vi "OSA_example_acquisition.vi"() -> ()   [LabVIEW 2010]
doc: "Simple example GUI for single asynchronous acquisition of spectrum with datareduction plotting functions. \n\nWhen creating custom dataacquisition applications displaying data; copy the graphs in this example, create corresponding graph references and connect to the init vi, see example diagram."
uses:
  _OSA_class/typeDef/resolution.ctl
  _OSA_class/typeDef/sensitivityMode.ctl
  _misc/Thorlabs_FTS_misc.llb/channels_table.ctl
  _misc/Thorlabs_FTS_misc.llb/channelType_spectrum.ctl
  _OSA_class/misc_examples/example_action.ctl
  _misc/Thorlabs_FTS_misc.llb/OSA_virtualModel.ctl
  _misc/Thorlabs_FTS_misc.llb/OSA_virtualSource_RS.ctl
  _OSA_class/typeDef/acq_dataType.ctl
  _OSA_class/OSA.lvclass
  OSA20X_misc.lvlib
panel:
  in  "virtual OSA":bool
  in  "spectrum channel type":T1
  in  "channels":T2
  in  "ZOOM OUT BUTTON":bool
  in  "PANE RIGHT":bool
  in  "PANE LEFT":bool
  in  "ZOOM RESTORE":bool
  in  "ZOOM IN BUTTON":bool
  in  "single acq butt":bool
  out "Intensity Graph spectrum":i32[][](graph)
  in  "sensitivity":T3=3 items=["low", "medium low", "medium high", "high"]
  in  "exit butt":bool
  in  "resolution":T4 items=["low", "high"]
  out "waveNrMax":sgl format="%.2f"
  out "waveNrMin":sgl format="%.2f"
  out "OSA":string
  # "Right click to autoscale Y"
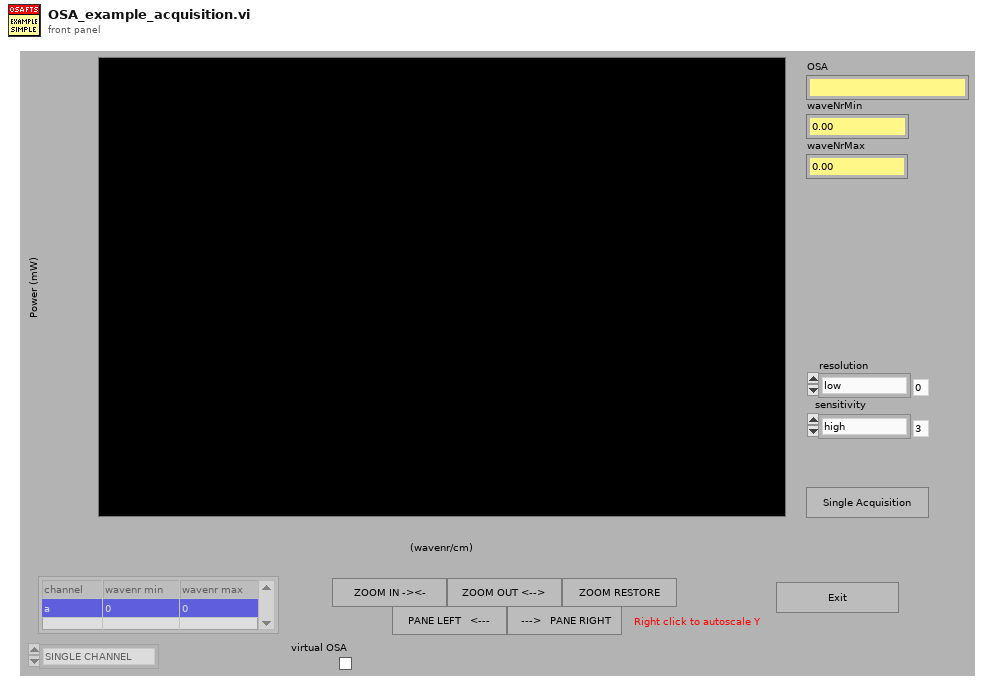
[diagram p1: front panel]
types:
  T1 = typedef "OSA20X_misc.lvlib/channelType_spectrum.ctl" = enum16{"SINGLE CHANNEL", "STICHED"}
  T2 = typedef "OSA20X_misc.lvlib/channels_table.ctl" = i32
  T3 = typedef "OSA.lvclass/sensitivityMode.ctl" = u16
  T4 = typedef "OSA.lvclass/resolution.ctl" = u16
  T5 = typedef "OSA20X_misc.lvlib/OSA_virtualSource_RS.ctl" = enum16{"VIRTUAL_REDSTONE_SOURCE_UNKNOWN", "VIRTUAL_REDSTONE_SOURCE_LLD_DFB_1530", "VIRTUAL_REDSTONE_SOURCE_SLD_1550nm", "VIRTUAL_REDSTONE_SOURCE_LASER_4600nm", "VIRTUAL_REDSTONE_SOURCE_BLACKBODY1500K", "VIRTUAL_REDSTONE_SOURCE_BLACKBODY1500K_H2O"}
  T6 = cluster{"OSA200":cluster{"waveCenter (nm)":dbl, "FWHM (nm)":dbl, "peakAmplitude":dbl}, "OSA300":T5}
  T7 = typedef "OSA20X_misc.lvlib/OSA_virtualModel.ctl" = enum16{"OSA201", "OSA201C", "OSA202", "OSA202C", "OSA203", "OSA203B", "OSA203C", "OSA205", "OSA205C", "REDSTONE301", "REDSTONE305"}
  T8 = typedef "OSA.lvclass/example_action.ctl" = enum16{"init", "user", "channel", "resolution set", "sensitivity set", "getSpectrum", "plotSpectrum"}
  T9 = cluster{"sensitivity ":refnum<vi>, "resolution":refnum<vi>, "channels":refnum<vi>, "spectrum channel type":refnum<vi>, "single acq butt":refnum<vi>}
  T10 = typedef "OSA.lvclass/acq_dataType.ctl" = enum16{"none", "interferogram", "spectrum"}
  T11 = enum8{"Enabled", "Disabled", "Disabled and Grayed Out"}
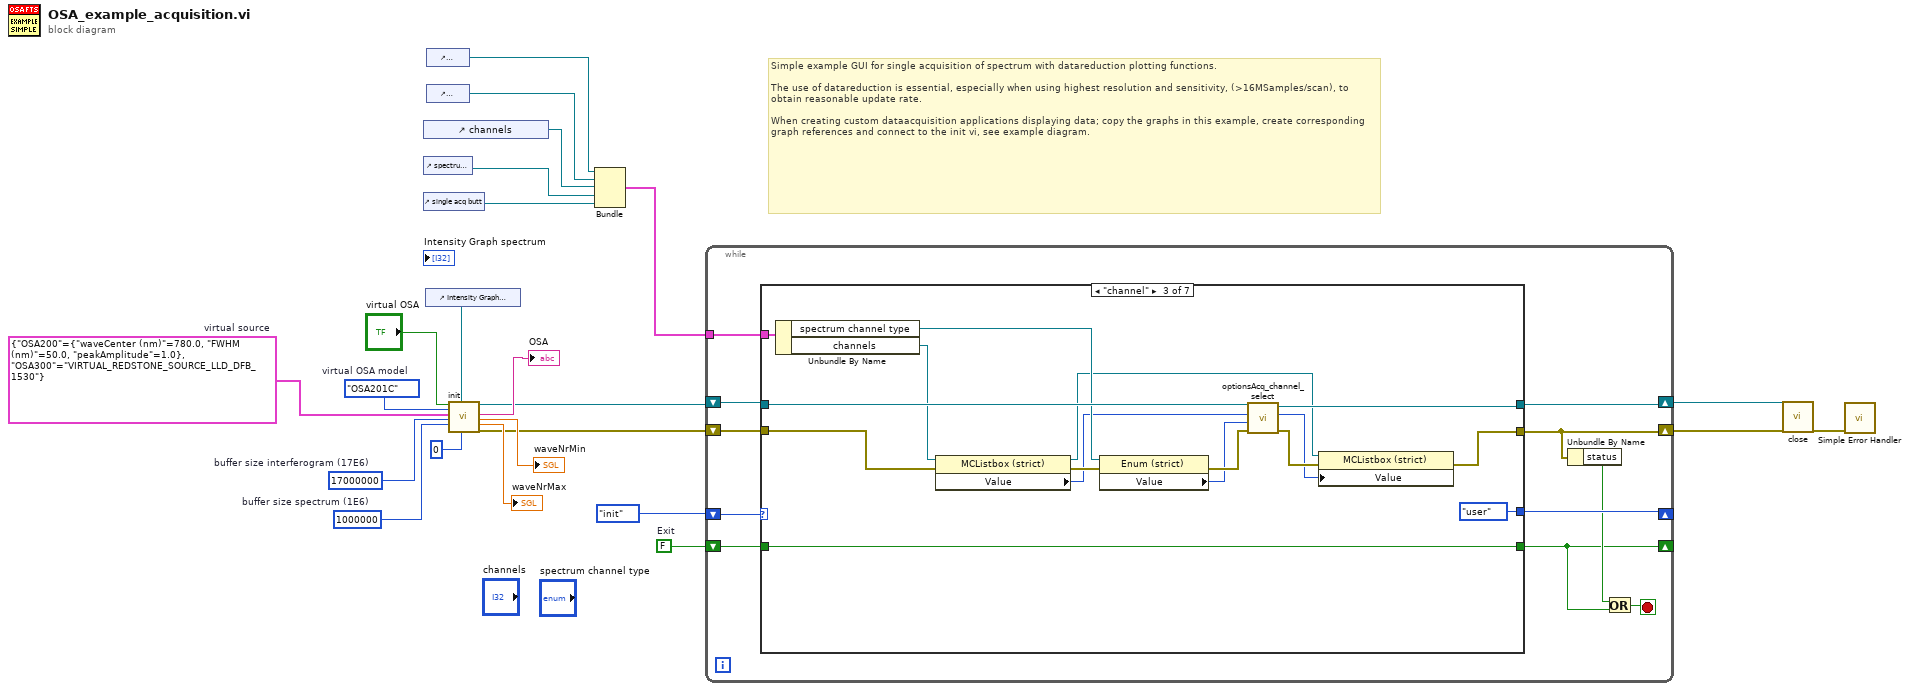
[diagram p0: block diagram]
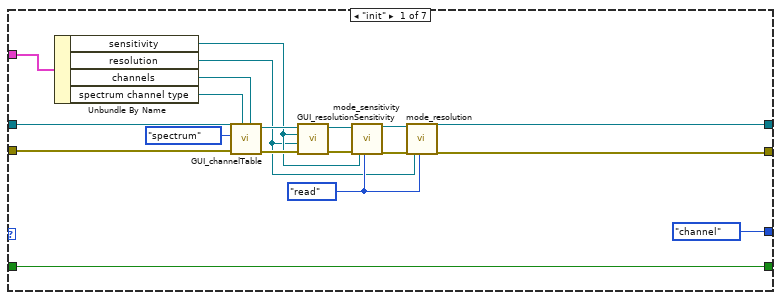
[diagram p2: hidden frame]
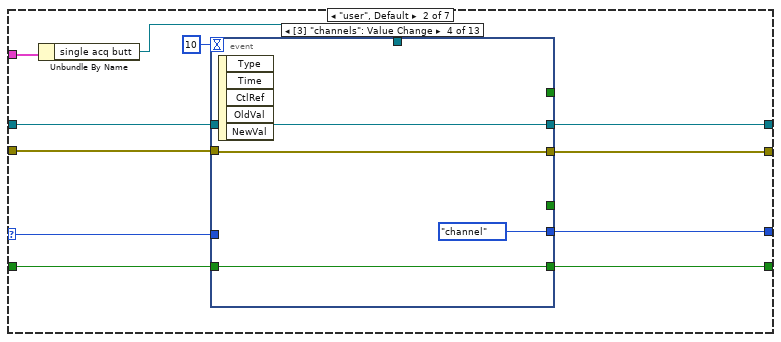
[diagram p3: hidden frame]
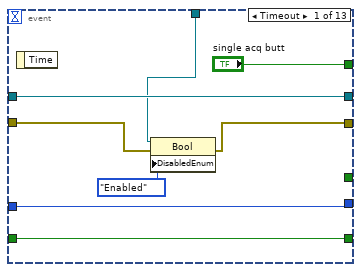
[diagram p4: hidden frame]
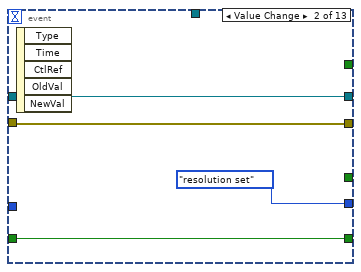
[diagram p5: hidden frame]
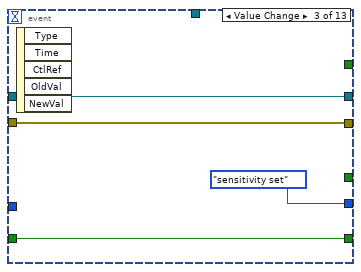
[diagram p6: hidden frame]
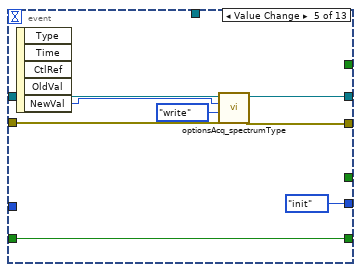
[diagram p7: hidden frame]
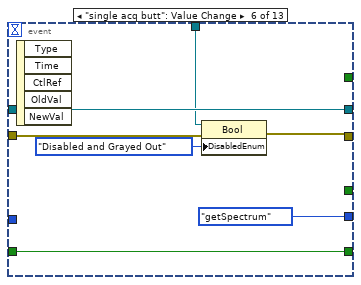
[diagram p8: hidden frame]
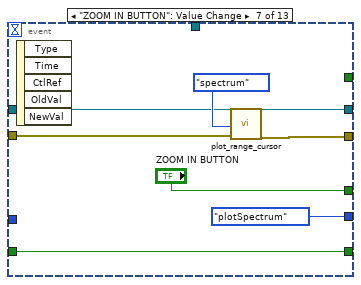
[diagram p9: hidden frame]
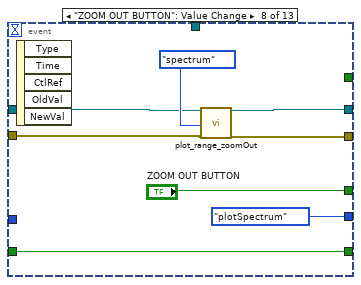
[diagram p10: hidden frame]
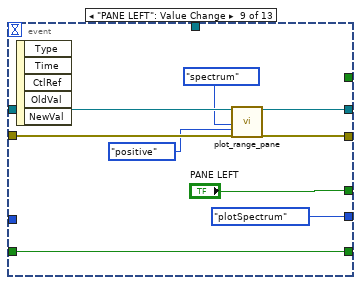
[diagram p11: hidden frame]
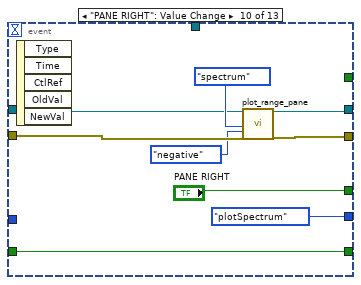
[diagram p12: hidden frame]
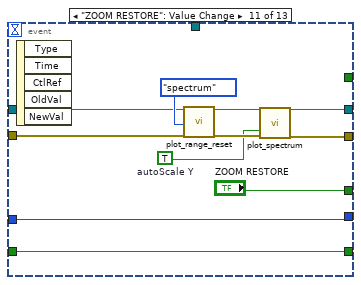
[diagram p13: hidden frame]
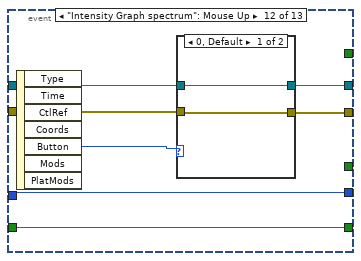
[diagram p14: hidden frame]
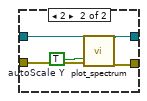
[diagram p15: hidden frame]
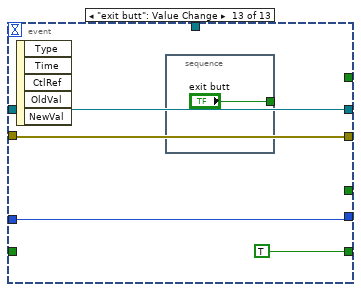
[diagram p16: hidden frame]
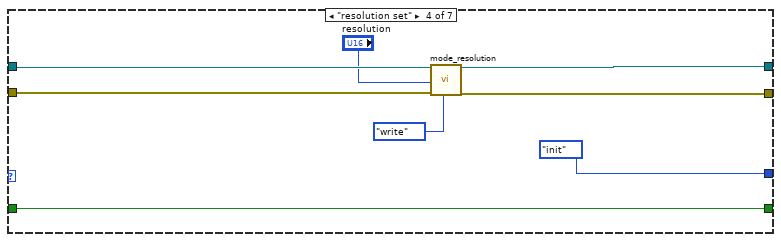
[diagram p17: hidden frame]
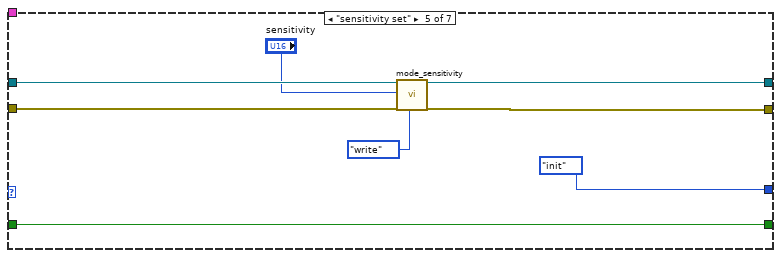
[diagram p18: hidden frame]
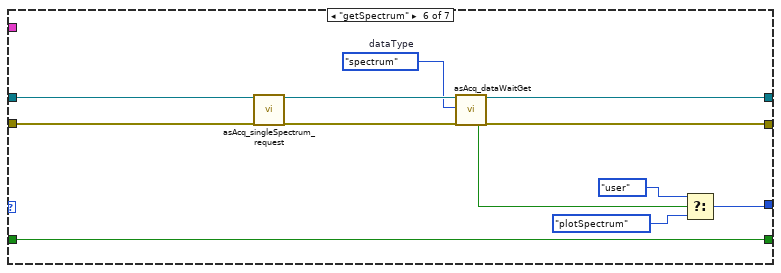
[diagram p19: hidden frame]
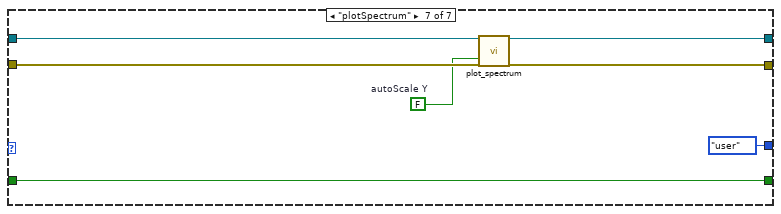
[diagram p20: hidden frame]
diagram:
  w3 = T6 {"OSA200"={"waveCenter (nm)"=780.0, "FWHM (nm)"=50.0, "peakAmplitude"=1.0}, "OSA300"=enum."VIRTUAL_REDSTONE_SOURCE_LLD_DFB_1530"}  # virtual source
  w4 = OSA_virtualModel."OSA201C"  # virtual OSA model
  w13 = 1000000  # buffer size spectrum (1E6)
  w14 = 17000000  # buffer size interferogram (17E6)
  w19 = FALSE  # Exit
  # "Simple example GUI for single acquisition of spectrum with datareduction plotting functions. \n\nThe use of datareduction is essential, especially when using highest resolution and sensitivity, (>16MSamples/scan), to obtain reasonable update rate.\n\nWhen creating custom dataacquisition applications displaying data; copy the graphs in this example, create corresponding graph references and connect to the init vi, see example diagram."
  n1 = control-ref of="channels"() -> (w11:refnum<vi>)
  n2 = control-ref of="spectrum channel type"() -> (w8:refnum<vi>)
  n3 = control-ref of="single acq butt"() -> (w10:refnum<vi>)
  n4 = control-ref of="Intensity Graph spectrum"() -> (w17:refnum<vi>)
  n5 = control-ref of="sensitivity"() -> (w6:refnum<vi>)
  n6 = control-ref of="resolution"() -> (w7:refnum<vi>)
  n7 = call "init.vi"("virtual OSA"="virtual OSA", "virtual OSA model"=w4, "virtual source"=w3, "buffer size interferogram (17E6)"=w14, "buffer size spectrum (1E6)"=w13, "Graph Spectrum"=w17, "spectrIdx"=u16 0) -> ("duplicate reference"=w2:refnum<class "OSA.lvclass">, "spectrometer"=→"OSA":string, "waveNrMin"=→"waveNrMin":sgl, "waveNrMax"=→"waveNrMax":sgl, "error out"=w16:errorcluster)  [unwired: 8 in]
  n8 = Bundle("sensitivity"=w6, "resolution"=w7, "channels"=w11, "spectrum channel type"=w8, "single acq butt"=w10) -> (w9:T9)  [unwired: 1 in]
  n9 = while {
    shift-right: [w30] -> w15
    shift-left: w16 -> [w34]
    shift-right: [w32] -> _
    shift-left: example_action."init" ("action") -> [w33]
    shift-right: [w27] -> _
    shift-left: w19 -> [w31]
    tunnel: w9 -> [w26]
    shift-right: [w24] -> w1
    shift-left: w2 -> [w25]
    stop <- w28 stop-if-true
    n10 = case shown="\"channel\"" w33 {
      selector: w33 -> [_ w62 _ _ _ _ _]
      tunnel: w34 -> [w50 w59 w176 w187 w195 w206 w214]
      tunnel: [example_action."channel" ("action") w63 example_action."user" ("action") example_action."init" ("action") example_action."init" ("action") w198 example_action."user" ("action")] -> w32
      tunnel: [w38 w58 w165 w185 w192 w202 w213] -> w30
      tunnel: w31 -> [w52 w61 w164 w184 w191 w207 w209]
      tunnel: [w52 w60 w164 w184 w191 w207 w209] -> w27
      tunnel: w25 -> [w51 w56 w178 w183 w194 w205 w211]
      tunnel: [w37 w57 w177 w182 w193 w201 w212] -> w24
      tunnel: w26 -> [w49 w55 w175 _ _ _ _]
      frame "init" {
        w39 = enum16{"read", "write"}."read" ("read/write")
        n11 = Unbundle By Name(w49) -> ("sensitivity"=w36:refnum<vi>, "resolution"=w35:refnum<vi>, "channels"=w47:refnum<vi>, "spectrum channel type"=w48:refnum<vi>)
        n12 = call "GUI_channelTable.vi"("ref channels table"=w47, "ref spectrum channel type"=w48, "error in (no error)"=w50, "dataType"=acq_dataType."spectrum", "Thorlabs_OSA_64 in"=w51) -> ("error out"=w45:errorcluster, "Thorlabs_OSA_64 out"=w44:refnum<class "OSA.lvclass">)  [unwired: 5 in]
        n13 = call-dynamic "GUI_resolutionSensitivity.vi"("error in (no error)"=w45, "resolution ref"=w35, "sensitivity ref"=w36, "Thorlabs_OSA_64 in"=w44) -> ("error out"=w43:errorcluster, "Thorlabs_OSA_64 out"=w42:refnum<class "OSA.lvclass">)  [unwired: 6 in]
        n14 = call-dynamic "mode_sensitivity.vi"("reference"=w42, "error in (no error)"=w43, "ctrl ref"=w36, "read/write"=w39) -> ("duplicate reference"=w41:refnum<class "OSA.lvclass">, "error out"=w40:errorcluster)  [unwired: 13 in, 1 out]
        n15 = call-dynamic "mode_resolution.vi"("reference"=w41, "error in (no error)"=w40, "ctrl ref"=w35, "read/write"=w39) -> ("duplicate reference"=w37:refnum<class "OSA.lvclass">, "error out"=w38:errorcluster)  [unwired: 12 in, 2 out]
      }
      frame "user", Default {
        n16 = Unbundle By Name(w55) -> ("single acq butt"=w54:refnum<vi>)
        n17 = event shown="[3] \"channels\": Value Change" {
          selector: _ -> [_ _ _ _ _ _ _ _ _ _ _ _ _]
          dyn-events: _ -> [_ _ _ _ _ _ _ _ _ _ _ _ _]
          timeout: 10 -> [_ _ _ _ _ _ _ _ _ _ _ _ _]
          tunnel: [w72 example_action."resolution set" ("action") example_action."sensitivity set" ("action") example_action."channel" ("action") example_action."init" ("action") example_action."getSpectrum" ("action") example_action."plotSpectrum" ("action") example_action."plotSpectrum" ("action") example_action."plotSpectrum" ("action") example_action."plotSpectrum" ("action") w140 w147 w161] -> w63
          tunnel: w62 -> [w72 _ _ _ _ _ _ _ _ _ w140 w147 w161]
          tunnel: w61 -> [w71 w75 w77 w81 w91 w98 w101 w109 w117 w126 w144 w146 _]
          tunnel: [w71 w75 w77 w81 w91 w98 w101 w109 w117 w126 w144 w146 TRUE ("abort")] -> w60
          tunnel: w59 -> [w69 w73 w78 w82 w90 w96 w106 w115 w124 w130 w142 w148 w159]
          tunnel: [w68 w73 w78 w82 w89 w95 w105 w114 w123 w131 w139 w150 w159] -> w58
          tunnel: [w70 w74 w79 w83 w88 w97 w104 w111 w122 w132 w138 w151 w160] -> w57
          tunnel: w56 -> [w70 w74 w79 w83 w87 w97 w103 w112 w121 w129 w141 w149 w160]
          tunnel: w54 -> [w67 _ _ _ _ w93 _ _ _ _ _ _ _]
          tunnel: ["single acq butt" _ _ _ _ _ _ _ _ _ _ _ _] -> _
          tunnel: [_ _ _ _ _ _ "ZOOM IN BUTTON" "ZOOM OUT BUTTON" "PANE LEFT" "PANE RIGHT" "ZOOM RESTORE" _ _] -> _
          event Timeout {
            n18 = event-data() -> ()  [unwired: 1 in, 1 out]
            n19 = property class="Bool"(reference=w67, error in=w69, "DisabledEnum"=T11."Enabled" ("Disabled")) -> (error out=w68:errorcluster)  [unwired: 1 out]
          }
          event Value Change {
            n20 = event-data() -> ()  [unwired: 1 in, 5 out]
          }
          event Value Change {
            n21 = event-data() -> ()  [unwired: 1 in, 5 out]
          }
          event Value Change {
            n22 = event-data() -> ()  [unwired: 1 in, 5 out]
          }
          event Value Change {
            n23 = event-data() -> ("NewVal"=w85:T1)  [unwired: 1 in, 4 out]
            n24 = call-dynamic "optionsAcq_spectrumType.vi"("error in (no error)"=w90, "readWrite"=enum16{"read", "write"}."write", "spectrum channel type"=w85, "Thorlabs_OSA_64 in"=w87) -> ("error out"=w89:errorcluster, "Thorlabs_OSA_64 out"=w88:refnum<class "OSA.lvclass">)  [unwired: 5 in, 1 out]
          }
          event "single acq butt": Value Change {
            n25 = event-data() -> ()  [unwired: 1 in, 5 out]
            n26 = property class="Bool"(reference=w93, error in=w96, "DisabledEnum"=T11."Disabled and Grayed Out" ("Disabled")) -> (error out=w95:errorcluster)  [unwired: 1 out]
          }
          event "ZOOM IN BUTTON": Value Change {
            n27 = event-data() -> ()  [unwired: 1 in, 5 out]
            n28 = call "plot_range_cursor.vi"("reference"=w103, "dataType"=acq_dataType."spectrum", "error in (no error)"=w106) -> ("duplicate reference"=w104:refnum<class "OSA.lvclass">, "error out"=w105:errorcluster)  [unwired: 15 in]
          }
          event "ZOOM OUT BUTTON": Value Change {
            n29 = event-data() -> ()  [unwired: 1 in, 5 out]
            n30 = call "plot_range_zoomOut.vi"("reference"=w112, "dataType"=acq_dataType."spectrum", "error in (no error)"=w115) -> ("duplicate reference"=w111:refnum<class "OSA.lvclass">, "error out"=w114:errorcluster)  [unwired: 15 in]
          }
          event "PANE LEFT": Value Change {
            n31 = event-data() -> ()  [unwired: 1 in, 5 out]
            n32 = call "plot_range_pane.vi"("reference"=w121, "dataType"=acq_dataType."spectrum", "direction"=enum16{"positive", "negative"}."positive", "error in (no error)"=w124) -> ("duplicate reference"=w122:refnum<class "OSA.lvclass">, "error out"=w123:errorcluster)  [unwired: 14 in]
          }
          event "PANE RIGHT": Value Change {
            n33 = event-data() -> ()  [unwired: 1 in, 5 out]
            n34 = call "plot_range_pane.vi"("reference"=w129, "dataType"=acq_dataType."spectrum", "direction"=enum16{"positive", "negative"}."negative", "error in (no error)"=w130) -> ("duplicate reference"=w132:refnum<class "OSA.lvclass">, "error out"=w131:errorcluster)  [unwired: 14 in]
          }
          event "ZOOM RESTORE": Value Change {
            w135 = TRUE  # autoScale Y
            n35 = event-data() -> ()  [unwired: 1 in, 5 out]
            n36 = call "plot_range_reset.vi"("reference"=w141, "dataType"=acq_dataType."spectrum", "error in (no error)"=w142) -> ("duplicate reference"=w136:refnum<class "OSA.lvclass">, "error out"=w137:errorcluster)  [unwired: 15 in]
            n37 = call "plot_spectrum.vi"("reference"=w136, "autoScale Y"=w135, "error in (no error)"=w137) -> ("duplicate reference"=w138:refnum<class "OSA.lvclass">, "error out"=w139:errorcluster)  [unwired: 15 in]
          }
          event "Intensity Graph spectrum": Mouse Up {
            n38 = event-data() -> ("Button"=w145:u16)  [unwired: 1 in, 6 out]
            n39 = case shown="0, Default" w145 {
              tunnel: [w153 w157] -> w151
              tunnel: [w152 w156] -> w150
              tunnel: w149 -> [w153 w155]
              tunnel: w148 -> [w152 w154]
              frame 0, Default {
              }
              frame 2 {
                w158 = TRUE  # autoScale Y
                n40 = call "plot_spectrum.vi"("reference"=w155, "autoScale Y"=w158, "error in (no error)"=w154) -> ("duplicate reference"=w157:refnum<class "OSA.lvclass">, "error out"=w156:errorcluster)  [unwired: 15 in]
              }
            }
          }
          event "exit butt": Value Change {
            n41 = event-data() -> ()  [unwired: 1 in, 5 out]
            n42 = stacked-sequence {
              tunnel: ["exit butt"] -> _
              frame #0 {
              }
            }
          }
        }
      }
      frame "channel" {
        n43 = Unbundle By Name(w175) -> ("spectrum channel type"=w172:refnum<vi>, "channels"=w174:refnum<vi>)
        n44 = property class="MCListbox (strict)"(reference=w174, error in=w176) -> (reference out=w167:refnum<vi>, error out=w173:errorcluster, "Value"=w171:i32)
        n45 = property class="Enum (strict)"(reference=w172, error in=w173) -> (error out=w170:errorcluster, "Value"=w169:enum16{"SINGLE CHANNEL", "STICHED"})  [unwired: 1 out]
        n46 = call-dynamic "optionsAcq_channel_select.vi"("error in (no error)"=w170, "channelType_spectrum"=w169, "channel DUT (index)"=w171, "Thorlabs_OSA_64 in"=w178) -> ("error out"=w168:errorcluster, "channel DUT out"=w166:i32, "Thorlabs_OSA_64 out"=w177:refnum<class "OSA.lvclass">)  [unwired: 5 in]
        n47 = property class="MCListbox (strict)"(reference=w167, error in=w168, "Value"=w166) -> (error out=w165:errorcluster)  [unwired: 1 out]
      }
      frame "resolution set" {
        n48 = call-dynamic "mode_resolution.vi"("reference"=w183, "resolution"="resolution", "error in (no error)"=w187, "read/write"=enum16{"read", "write"}."write") -> ("duplicate reference"=w182:refnum<class "OSA.lvclass">, "error out"=w185:errorcluster)  [unwired: 12 in, 2 out]
      }
      frame "sensitivity set" {
        n49 = call-dynamic "mode_sensitivity.vi"("reference"=w194, "sensitivity"="sensitivity", "error in (no error)"=w195, "read/write"=enum16{"read", "write"}."write") -> ("duplicate reference"=w193:refnum<class "OSA.lvclass">, "error out"=w192:errorcluster)  [unwired: 13 in, 1 out]
      }
      frame "getSpectrum" {
        w196 = acq_dataType."spectrum"  # dataType
        n50 = call "asAcq_singleSpectrum_request.vi"("reference"=w205, "error in (no error)"=w206) -> ("duplicate reference"=w204:refnum<class "OSA.lvclass">, "error out"=w203:errorcluster)  [unwired: 16 in]
        n51 = call-dynamic "asAcq_dataWaitGet.vi"("reference"=w204, "dataType"=w196, "error in (no error)"=w203) -> ("timeOut"=w197:bool, "duplicate reference"=w201:refnum<class "OSA.lvclass">, "error out"=w202:errorcluster)  [unwired: 13 in, 1 out]
        n52 = Select(t=example_action."user" ("action"), s=w197, f=example_action."plotSpectrum" ("action")) -> (s? t:f=w198:T8)
      }
      frame "plotSpectrum" {
        w208 = FALSE  # autoScale Y
        n53 = call "plot_spectrum.vi"("reference"=w211, "autoScale Y"=w208, "error in (no error)"=w214) -> ("duplicate reference"=w212:refnum<class "OSA.lvclass">, "error out"=w213:errorcluster)  [unwired: 15 in]
      }
    }
    n54 = Unbundle By Name(w30) -> ("status"=w29:bool)
    n55 = Or(x=w29, y=w27) -> (x .or. y?=w28:bool)
  }
  n56 = call "close.vi"("reference"=w1, "error in (no error)"=w15) -> ("error out"=w23:errorcluster)  [unwired: 17 in]
  n57 = call <vilib>:"Simple Error Handler.vi"("error in (no error)"=w23) -> ()  [unwired: 4 in, 5 out]
